vi "restInitHTTP.vi"(8 "error in (no error)":errorcluster, 11 "access token":string) -> (0 "error out":errorcluster, 3 "Refnum out":T1)   [LabVIEW 2018, in "HASS-LV-WS_integration.lvlib"]
uses:
  <vilib>/httpClient/ClientHandle.ctl
  HASS-LV-WS_integration.lvlib
  <vilib>/httpClient/LabVIEWHTTPClient.lvlib
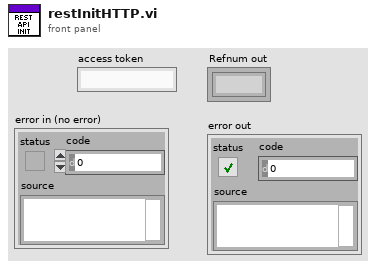
[diagram p1: front panel]
types:
  T1 = typedef "LabVIEWHTTPClient.lvlib/ClientHandle.ctl" = refnum<k1>
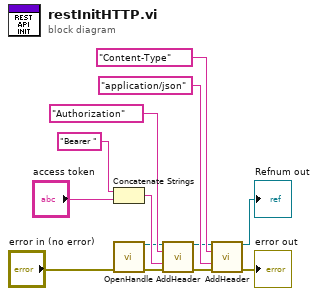
[diagram p0: block diagram]
diagram:
  n1 = Concatenate Strings("Bearer " ("string"), "access token") -> (w11:string)
  n2 = call <vilib>:"OpenHandle.vi"("error in (no error)"="error in (no error)") -> ("client handle out"=w2:T1, "error out"=w3:errorcluster)  [unwired: 13 in]
  n3 = call <vilib>:"AddHeader.vi"("client handle"=w2, "header"="Authorization", "value"=w11, "error in (no error)"=w3) -> ("client handle out"=w4:T1, "error out"=w5:errorcluster)  [unwired: 10 in]
  n4 = call <vilib>:"AddHeader.vi"("client handle"=w4, "header"="Content-Type", "value"="application/json", "error in (no error)"=w5) -> ("client handle out"=→"Refnum out":T1, "error out"=→"error out":errorcluster)  [unwired: 10 in]
